vi "Write FPGA VI Reference Out.vi"(8 "error in (no error)":errorcluster, 10 "FPGA VI Reference Out":refnum<k20>, 11 "FpgaRunner in":refnum<class "FpgaRunner.lvclass">) -> (0 "error out":errorcluster, 3 "FpgaRunner out":refnum<class "FpgaRunner.lvclass">)   [LabVIEW 2020, in "FpgaRunner.lvclass"]
uses:
  FpgaRunner.lvclass
  FpgaRunner.lvclass/FpgaRunner.ctl
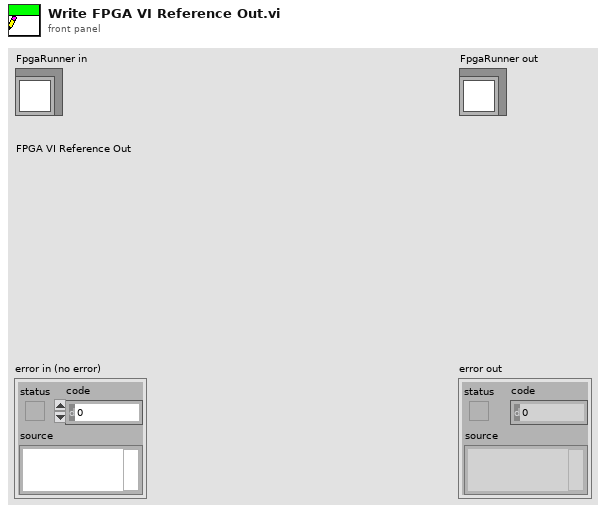
[diagram p1: front panel]
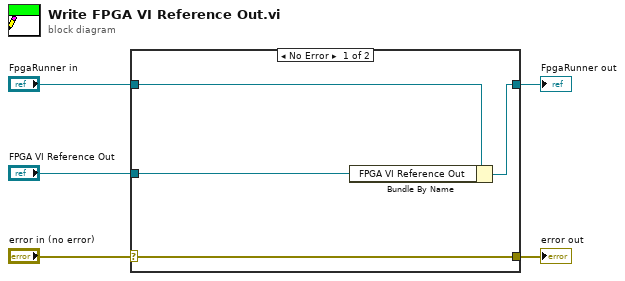
[diagram p0: block diagram]
diagram:
  n1 = case shown="No Error" "error in (no error)" {
    selector: "error in (no error)" -> [w9 w10]
    tunnel: [w9 w10] -> w4
    tunnel: [w7 w11] -> w2
    tunnel: "FpgaRunner in" -> [w8 w11]
    tunnel: "FPGA VI Reference Out" -> [w6 _]
    frame No Error {
      n2 = Bundle By Name(cluster=w8, "FPGA VI Reference Out"=w6) -> (w7:refnum<class "FpgaRunner.lvclass">)
    }
    frame Error {
    }
  }
  "error out" <- w4
  "FpgaRunner out" <- w2
